vi "XY Graph Get Plot Data & Info.vi"(0 "Destination Graph":refnum<vi>, 5 "Original Graph":refnum<vi>, 7 "Original Plot Idx":i32=-1, 11 "Error In":errorcluster, 12 "Plot Style in":T2={"PlotIndex"=0, "BarPlotStyle"=0, "DigitalLineStyle"=1, "TransitionLocation"=2, "TransitionType"=0, "FillTo"=-1, "FillPointColor"=16777222, "LabelFormat"=3, "LineStyle"=0, "LineWidth"=1, "PlotColor"=16777222, "PlotInterpolation"=2, "PlotName"="", "PointStyle"=0, "Visible"=TRUE, "XScaleIdx"=0, "YScaleIdx"=0, "AntiAliased"=TRUE}, 13 "Plot in":T1, 14 "Graph Origin Name":string) -> (3 "Refnum based call":bool, 4 "VI Title Suffix":string, 6 "X Array":dbl[](array[numeric]), 8 "Y Array":dbl[](array[numeric]), 10 "Plot Style out":T2, 15 "Error Out":errorcluster)   [LabVIEW 2021, in "XY Graph Add-Ons.lvlib"]
uses:
  XY Graph Add-Ons.lvlib
  XY Graph Plot Properties.ctl
  XY Graph Plot Data.ctl
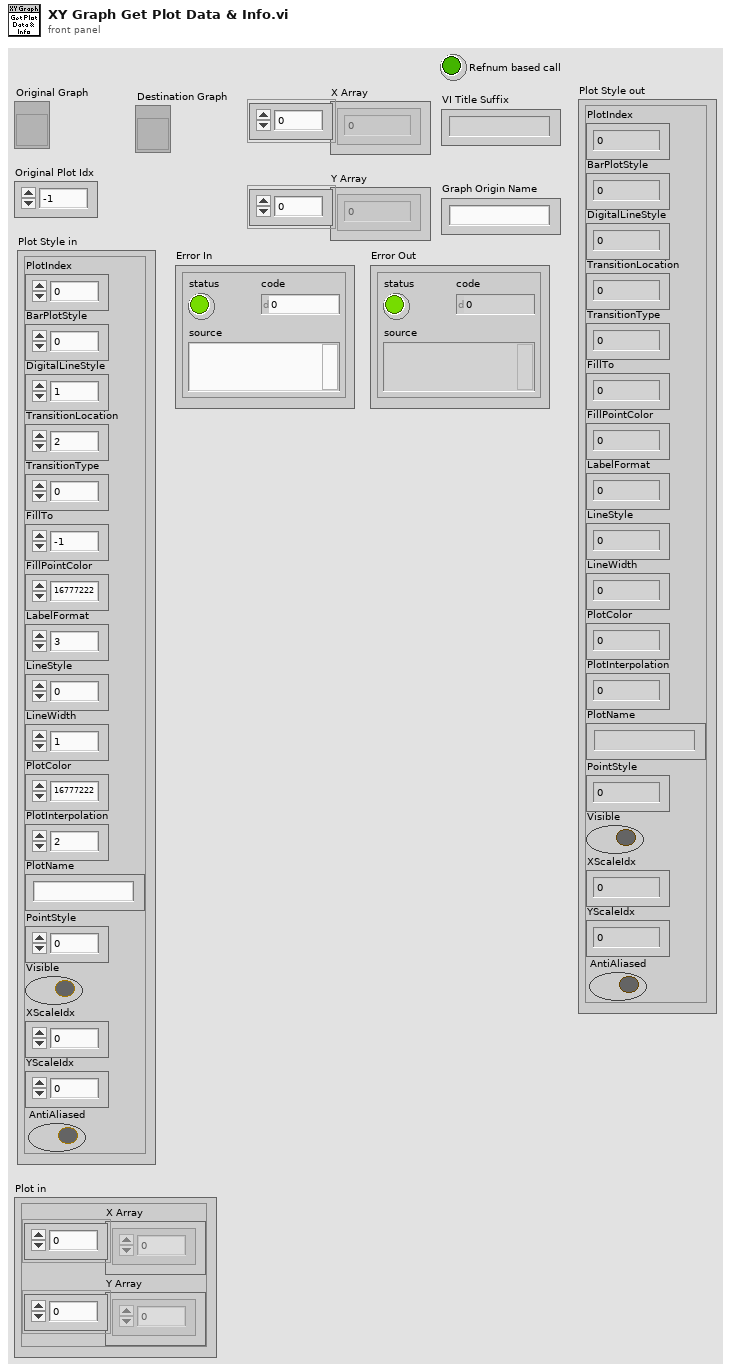
[diagram p1: front panel]
types:
  T1 = typedef "XY Graph Add-Ons.lvlib/XY Graph Plot Data.ctl" = cluster{"X Array":dbl[], "Y Array":dbl[]}
  T2 = typedef "XY Graph Add-Ons.lvlib/XY Graph Plot Properties.ctl" = cluster{"PlotIndex":i32, "BarPlotStyle":u8, "DigitalLineStyle":u8, "TransitionLocation":u8, "TransitionType":u8, "FillTo":i16, "FillPointColor":u32, "LabelFormat":u8, "LineStyle":u8, "LineWidth":u8, "PlotColor":u32, "PlotInterpolation":u8, "PlotName":string, "PointStyle":u8, "Visible":bool, "XScaleIdx":u32, "YScaleIdx":u32, "AntiAliased":bool}
  T3 = typedef "XY Graph Add-Ons.lvlib/XY Graph Refnum.ctl" = refnum<vi>
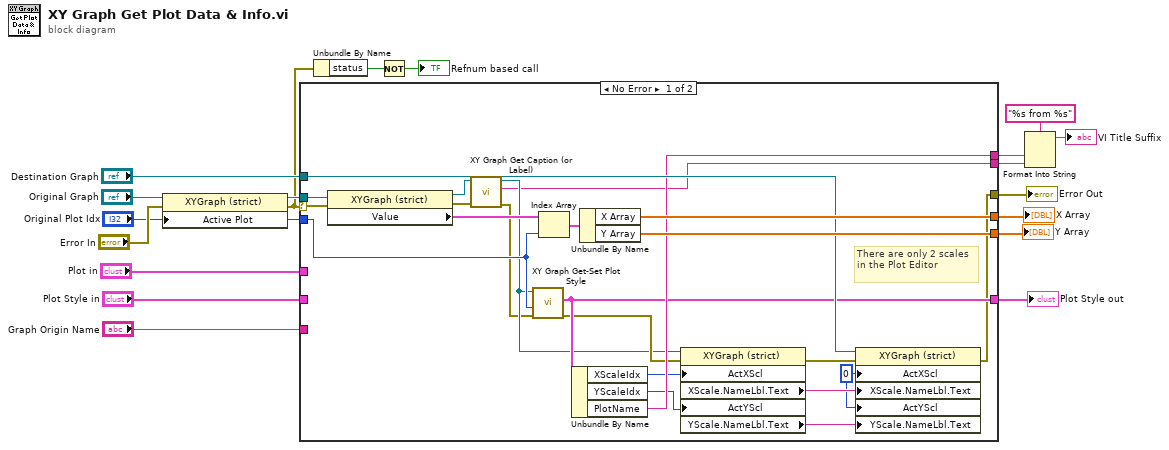
[diagram p0: block diagram]
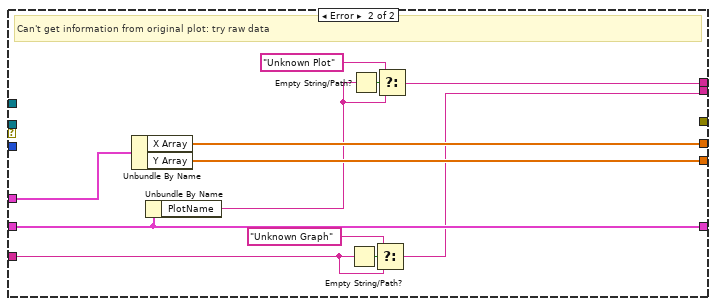
[diagram p2: hidden frame]
diagram:
  n1 = property class="XYGraph (strict)"(reference="Original Graph", error in="Error In", "Active Plot"="Original Plot Idx") -> (reference out=w12:refnum<vi>, error out=w3:errorcluster)
  n2 = case shown="No Error" w3 {
    selector: w3 -> [w26 _]
    tunnel: "Plot in" -> [_ w54]
    tunnel: [w39 w53] -> w17
    tunnel: [w38 w52] -> w16
    tunnel: "Plot Style in" -> [_ w51]
    tunnel: [w27 w51] -> w14
    tunnel: w12 -> [w42 _]
    tunnel: "Original Plot Idx" -> [w29 _]
    tunnel: [w24 _] -> w10
    tunnel: "Destination Graph" -> [w35 _]
    tunnel: [w33 w49] -> w6
    tunnel: [w20 w46] -> w5
    tunnel: "Graph Origin Name" -> [_ w45]
    frame No Error {
      w28 = 0 ("Active X Scale")
      # "There are only 2 scales in the Plot Editor"
      n3 = property class="XYGraph (strict)"(reference=w42, error in=w26) -> (reference out=w37:refnum<vi>, error out=w22:errorcluster, "Value"=w41:cluster{"X Array":dbl[], "Y Array":dbl[]}[])
      n4 = call "XY Graph Get Caption (or Label).vi"("error in (no error)"=w22, "XY Graph in"=w37) -> ("error out"=w21:errorcluster, "Caption (or Label) Text"=w20:string, "XY Graph out"=w23:T3)  [unwired: 7 in]
      n5 = call "XY Graph Get-Set Plot Style.vi"("Error In"=w21, "Plot Index"=w29, "XYGraph in"=w23) -> ("Error Out"=w25:errorcluster, "Plot Style out"=w27:T2)  [unwired: 5 in, 2 out]
      n6 = Index Array(array=w41, index=w29) -> (element=w40:cluster{"X Array":dbl[], "Y Array":dbl[]})
      n7 = Unbundle By Name(w27) -> ("XScaleIdx"=w31:u32, "YScaleIdx"=w30:u32, "PlotName"=w33:string)
      n8 = Unbundle By Name(w40) -> ("X Array"=w39:dbl[], "Y Array"=w38:dbl[])
      n9 = property class="XYGraph (strict)"(reference=w23, error in=w25, "ActXScl"=w31, "ActYScl"=w30) -> (error out=w34:errorcluster, "XScale.NameLbl.Text"=w32:string, "YScale.NameLbl.Text"=w36:string)  [unwired: 1 out]
      n10 = property class="XYGraph (strict)"(reference=w35, error in=w34, "ActXScl"=w28, "XScale.NameLbl.Text"=w32, "ActYScl"=w28, "YScale.NameLbl.Text"=w36) -> (error out=w24:errorcluster)  [unwired: 1 out]
    }
    frame Error {
      # "Can't get information from original plot: try raw data"
      n11 = Unbundle By Name(w54) -> ("X Array"=w53:dbl[], "Y Array"=w52:dbl[])
      n12 = Unbundle By Name(w51) -> ("PlotName"=w48:string)
      n13 = Empty String/Path?(string/path=w45) -> (empty?=w47:bool)
      n14 = Empty String/Path?(string/path=w48) -> (empty?=w50:bool)
      n15 = Select(t="Unknown Graph", s=w47, f=w45) -> (s? t:f=w46:string)
      n16 = Select(t="Unknown Plot", s=w50, f=w48) -> (s? t:f=w49:string)
    }
  }
  "Plot Style out" <- w14
  "Y Array" <- w16
  "X Array" <- w17
  "Error Out" <- w10
  n17 = Unbundle By Name(w3) -> ("status"=w2:bool)
  n18 = Not(x=w2) -> (.not. x?=→"Refnum based call":bool)
  n19 = Format Into String(format string="%s from %s", w6, w5) -> (resulting string=→"VI Title Suffix":string)  [unwired: 2 in, 1 out]
